vi "createTelemetryForceActuatorStatus.vi"(8 "error in (no error)":errorcluster, 11 "UserEvents in":refnum<class "UserEvents.lvclass">) -> (0 "error out":errorcluster, 3 "UserEvents out":refnum<class "UserEvents.lvclass">)   [LabVIEW 2016, in "UserEvents.lvclass"]
uses:
  UserEvents.lvclass
  DataTypes/Topics/TelemetryForceActuatorStatus.ctl
  DataTypes/Topics/Parts/Timestamp.ctl
  UserEvents.lvclass/UserEvents.ctl
  DataTypes/Topics/M1M3SupportTopics.lvlib
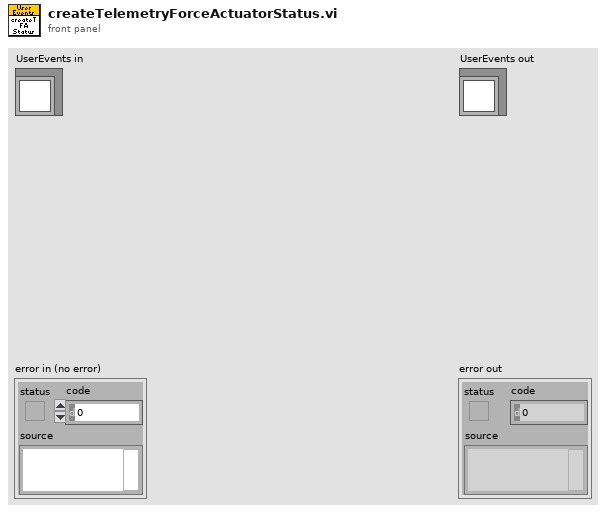
[diagram p1: front panel]
types:
  T1 = typedef "M1M3SupportTopics.lvlib/TelemetryForceActuatorStatus.ctl" = cluster{"Timestamp":T2, "Mode":u8[], "MajorFault":bool[], "MinorFault":bool[], "FaultOverridden":bool[], "DCAFault":bool[], "WatchdogReset":bool[], "BrownoutDetected":bool[], "EventTrapReset":bool[], "MotorPowerFault":bool[], "SSRPowerFault":bool[], "AUXPowerFault":bool[], "SMCPowerFault":bool[], "DCAOutputsEnabled":bool[], "DCAPowerFault":bool[], "DCAAmplifierAFault":bool[], "DCAAmplifierBFault":bool[], "DCAEventTrapReset":bool[]}
  T2 = typedef "M1M3SupportTopics.lvlib/Timestamp.ctl" = dbl
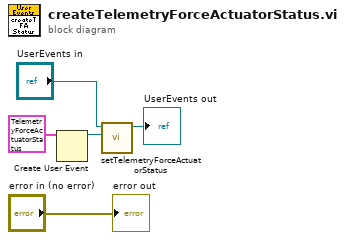
[diagram p0: block diagram]
diagram:
  n1 = Create User Event(user event datatype=T1 {"Timestamp"=0.0, "Mode"=[], "MajorFault"=[], "MinorFault"=[], "FaultOverridden"=[], "DCAFault"=[], "WatchdogReset"=[], "BrownoutDetected"=[], "EventTrapReset"=[], "MotorPowerFault"=[], "SSRPowerFault"=[], "AUXPowerFault"=[], "SMCPowerFault"=[], "DCAOutputsEnabled"=[], "DCAPowerFault"=[], "DCAAmplifierAFault"=[], "DCAAmplifierBFault"=[], "DCAEventTrapReset"=[]} ("TelemetryForceActuatorStatus")) -> (user event=w1:refnum<user-event>)  [unwired: 1 in, 1 out]
  n2 = call "setTelemetryForceActuatorStatus.vi"("TelemetryForceActuatorStatus"=w1, "UserEvents in"="UserEvents in") -> ("UserEvents out"=→"UserEvents out":refnum<class "UserEvents.lvclass">)  [unwired: 9 in]
  "error out" <- "error in (no error)"
